vi "ingest.tabular_set_channel_prefix.vi"(8 "error in":errorcluster, 11 "TabularIngestStaging in":refnum<class "TabularIngestStaging.lvclass">) -> (0 "error out":errorcluster, 3 "TabularIngestStaging out":refnum<class "TabularIngestStaging.lvclass">)   [LabVIEW 2020, in "TabularIngestStaging.lvclass"]
doc: "Adds a prefix to every channel name created from the ingested file."
uses:
  TabularIngestStaging.lvclass
  TabularIngestStaging.lvclass/TabularIngestStaging.ctl
  client.lvlib
panel:
  in  "prefix":string
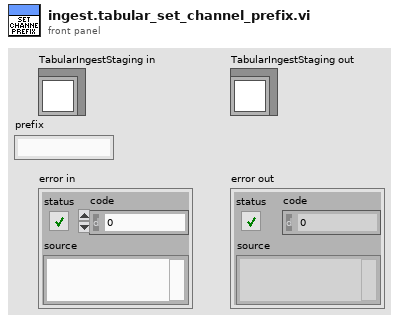
[diagram p1: front panel]
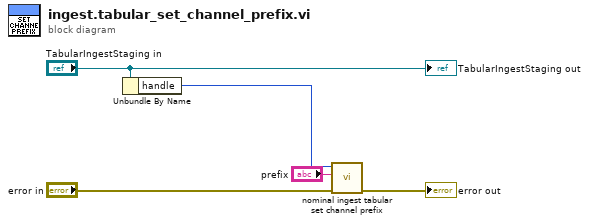
[diagram p0: block diagram]
diagram:
  n1 = Unbundle By Name("TabularIngestStaging in") -> ("handle"=w3:i32)
  n2 = call "nominal ingest tabular set channel prefix.vi"("error in (no error)"="error in", "prefix"="prefix", "staging"=w3) -> ("error out"=→"error out":errorcluster)  [unwired: 7 in, 1 out]
  "TabularIngestStaging out" <- "TabularIngestStaging in"
